vi "4-16 decoder.vi"() -> ()   [LabVIEW 2012]
panel:
  out "Boolean 4":bool
  out "Array":dbl[](array[numeric])
  in  "Boolean 3":bool
  in  "Boolean 2":bool
  in  "Boolean":bool
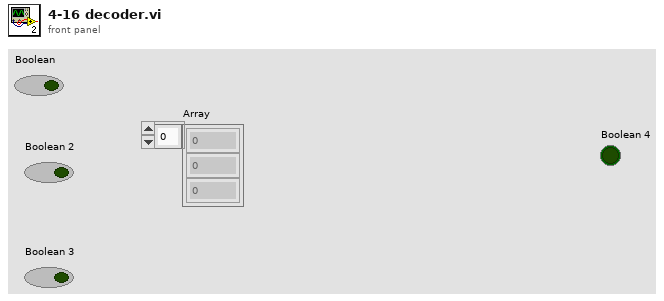
[diagram p1: front panel]
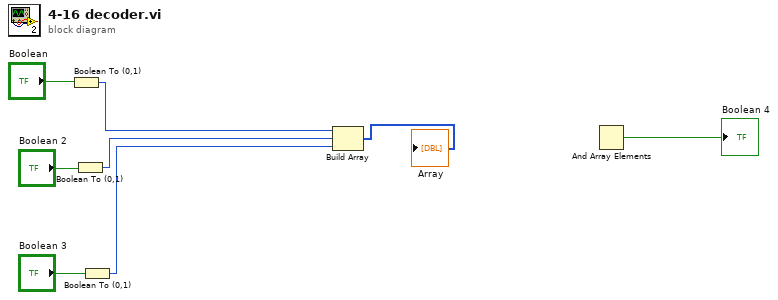
[diagram p0: block diagram]
diagram:
  n1 = Boolean To (0,1)(Boolean="Boolean") -> (0, 1=w5:i16)
  n2 = Boolean To (0,1)(Boolean="Boolean 2") -> (0, 1=w4:i16)
  n3 = Boolean To (0,1)(Boolean="Boolean 3") -> (0, 1=w3:i16)
  n4 = Build Array "Build Array"(w5, w4, w3) -> (→"Array":i16[])
  n5 = And Array Elements() -> (logical AND=→"Boolean 4":bool)  [unwired: 1 in]
